vi "SoundGen.vi"() -> ()   [LabVIEW 2017]
uses:
  <vilib>/sound2/lvsound2.llb/Sampling Mode.ctl
  <vilib>/sound2/lvsound2.llb/Sound Data Format.ctl
  <vilib>/sound2/lvsound2.llb/Sound Output Write (DBL).vi
  <vilib>/measure/NI_MABase.lvlib
panel:
  in  "amplitude 2":dbl=1.0 format="%0.2p"
  in  "frequency 2":dbl=10.0 format="%0.2p"
  in  "stop":bool
  in  "amplitude":dbl=1.0 format="%0.2p"
  in  "frequency":dbl=10.0 format="%0.2p"
  out "Waveform Graph":waveform(dbl)[](graph)
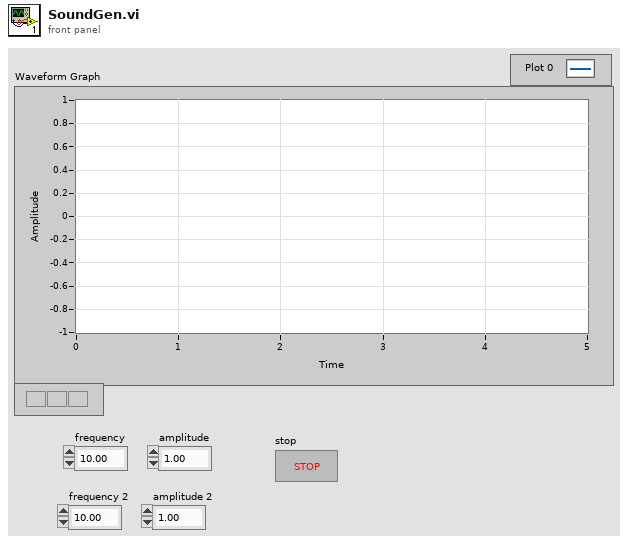
[diagram p1: front panel]
types:
  T1 = typedef "Sound Data Format.ctl" = cluster{"sample rate (S/s)":dbl, "number of channels":i32, "bits per sample":i32}
  T2 = typedef "Sampling Mode.ctl" = i32
  T3 = typedef "Sound Output Task ID.ctl" = u32
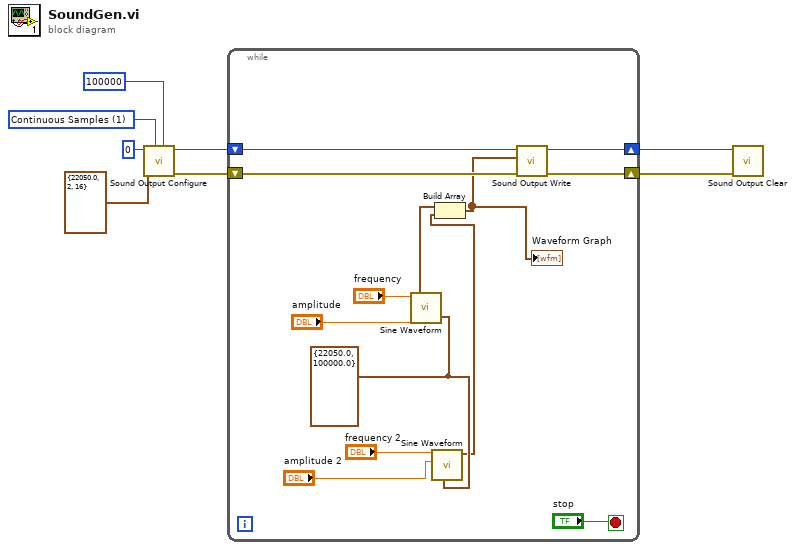
[diagram p0: block diagram]
diagram:
  w7 = T2 1 items=["Finite Samples", "Continuous Samples"] ("sample mode")
  n1 = call <vilib>:"Sound Output Configure.vi"("number of samples/ch"=100000, "sample mode"=w7, "sound format"=T1 {"sample rate (S/s)"=22050.0, "number of channels"=2, "bits per sample"=16}, "device ID"=u32 0) -> ("error out"=w4:errorcluster, "task ID"=w3:T3)  [unwired: 6 in]
  n2 = while {
    shift-right: [w15] -> w1
    shift-left: w4 -> [w21]
    shift-right: [w16] -> w2
    shift-left: w3 -> [w20]
    stop <- "stop" stop-if-true
    w11 = cluster{"Fs":dbl, "#s":dbl} {"Fs"=22050.0, "#s"=100000.0} ("sampling info")
    n3 = call <vilib>:"Sine Waveform.vi"("sampling info"=w11, "amplitude"="amplitude", "frequency"="frequency") -> ("signal out"=w17:waveform(dbl))  [unwired: 7 in, 1 out]
    n4 = call <vilib>:"Sine Waveform.vi"("sampling info"=w11, "amplitude"="amplitude 2", "frequency"="frequency 2") -> ("signal out"=w10:waveform(dbl))  [unwired: 7 in, 1 out]
    n5 = Build Array(w17, w10) -> (w9:waveform(dbl)[])
    "Waveform Graph" <- w9
    n6 = call-poly <vilib>:"Sound Output Write.vi"("error in (no error)"=w21, "data"=w9, "task ID"=w20) -> ("error out"=w15:errorcluster, "task ID out"=w16:T3)  [unwired: 7 in]
  }
  n7 = call <vilib>:"Sound Output Clear.vi"("error in (no error)"=w1, "task ID"=w2) -> ()  [unwired: 9 in, 1 out]
